vi "LogInfo.vi"(8 "error in (no error)":errorcluster, 10 "Info":string) -> (0 "error out":errorcluster)   [LabVIEW 2014, in "GCMLog.lvclass"]
uses:
  GCMLog.lvclass
  GCMLogGlobals.vi
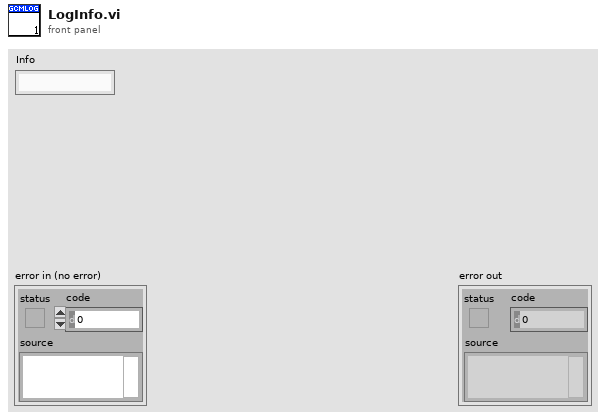
[diagram p1: front panel]
types:
  T1 = enum16{"open", "replace", "create", "open or create", "replace or create", "replace or create with confirmation"}
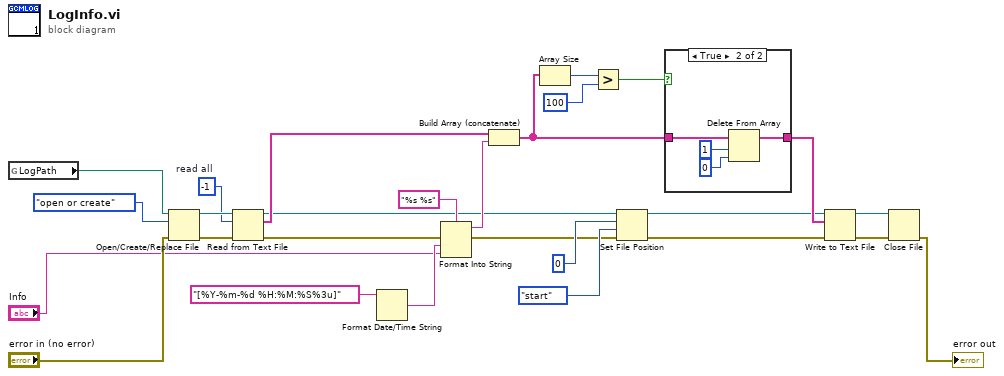
[diagram p0: block diagram]
diagram:
  w9 = -1  # read all
  n1 = global read "GCMLogGlobals.vi" "LogPath"() -> (w7:path)
  n2 = Open/Create/Replace File(file path (use dialog)=w7, error in="error in (no error)", operation (0:open)=T1."open or create") -> (refnum out=w22:refnum<file>, error out=w27:errorcluster)  [unwired: 3 in, 1 out]
  n3 = Read from Text File(file (use dialog)=w22, count=w9, error in=w27) -> (refnum out=w3:refnum<file>, text=w10:string[], error out=w16:errorcluster)  [unwired: 1 in, 1 out]
  n4 = Format Date/Time String(time format string (%c)="[%Y-%m-%d %H:%M:%S%3u]") -> (date/time string=w20:string)  [unwired: 2 in]
  n5 = Format Into String(format string="%s %s", error in=w16, w20, "Info") -> (resulting string=w15:string, error out=w4:errorcluster)  [unwired: 1 in]
  n6 = Build Array (concatenate)(w10, w15) -> (w12:string[])
  n7 = Array Size(array=w12) -> (size(s)=w14:i32)
  n8 = Greater?(x=w14, y=100) -> (0:w8:bool)
  n9 = Set File Position(offset (in bytes) (0)=i64 0, refnum=w3, from (0:start)=enum16{"start", "end", "current"}."start", error in=w4) -> (refnum out=w2:refnum<file>, error out=w1:errorcluster)
  n10 = case shown="True" w8 {
    tunnel: w12 -> [w28 w32]
    tunnel: [w28 w31] -> w11
    frame False {
    }
    frame True {
      n11 = Delete From Array(array=w32, length=1, index=0) -> (array with subset deleted=w31:string[])  [unwired: 1 out]
    }
  }
  n12 = Write to Text File(file (use dialog)=w2, text=w11, error in=w1) -> (refnum out=w21:refnum<file>, error out=w17:errorcluster)  [unwired: 1 in, 1 out]
  n13 = Close File(refnum=w21, error in=w17) -> (error out=→"error out":errorcluster)  [unwired: 1 out]
